vi "Get Plot at Mouse Click in Plot Area [CA].vi"(8 "error in (no error)":errorcluster, 10 "Mouse Click Coordinates":T1, 11 "XY Graph":refnum<vi>) -> (0 "error out":errorcluster, 1 "Plot Index":i32, 3 "XY Graph":refnum<vi>)   [LabVIEW 2021, in "Graphs.lvlib"]
uses:
  Graphs.lvlib
  <vilib>/Utility/miscctls.llb/LVPoint32TypeDef.ctl
panel:
  in  "Array of Complex Numbers":cdb[](array[numeric])
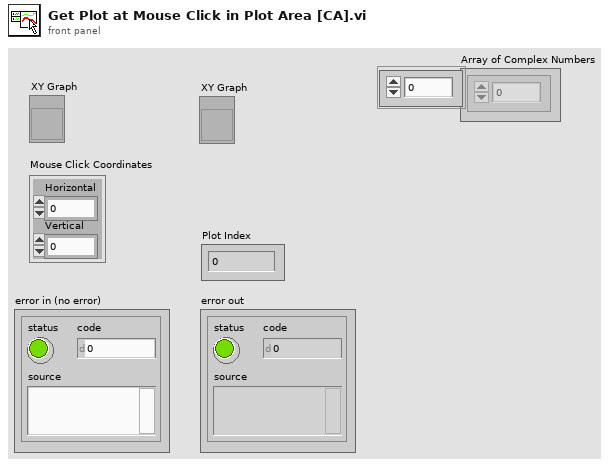
[diagram p1: front panel]
types:
  T1 = typedef "LVPoint32TypeDef.ctl" = cluster{"Horizontal":i32, "Vertical":i32}
  T2 = typedef "LVRectTypeDef.ctl" = cluster{"Left":i16, "Top":i16, "Right":i16, "Bottom":i16}
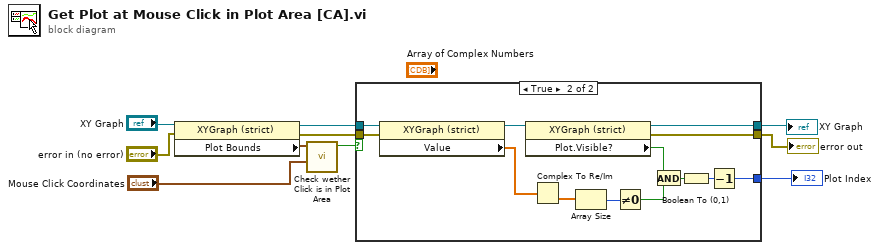
[diagram p0: block diagram]
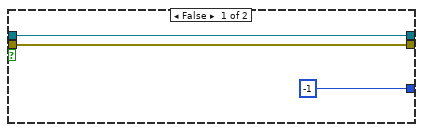
[diagram p2: hidden frame]
diagram:
  n1 = property class="XYGraph (strict)"(reference="XY Graph", error in="error in (no error)") -> (reference out=w6:refnum<vi>, error out=w7:errorcluster, "Plot Bounds"=w1:T2)
  n2 = call "Check wether Click is in Plot Area.vi"("Mouse Click Coordinates"="Mouse Click Coordinates", "Plot Bounds"=w1) -> ("Is in Plot Area?"=w8:bool)  [unwired: 8 in, 1 out]
  n3 = case shown="True" w8 {
    tunnel: w7 -> [w12 w22]
    tunnel: w6 -> [w13 w26]
    tunnel: [w13 w24] -> w5
    tunnel: [w12 w14] -> w4
    tunnel: [-1 ("Plot Index") w15] -> w3
    frame False {
    }
    frame True {
      n4 = property class="XYGraph (strict)"(reference=w26, error in=w22) -> (reference out=w25:refnum<vi>, "Value"=w23:cdb[])  [unwired: 1 out]
      n5 = property class="XYGraph (strict)"(reference=w25) -> (reference out=w24:refnum<vi>, error out=w14:errorcluster, "Plot.Visible?"=w19:bool)  [unwired: 1 in]
      n6 = Complex To Re/Im(x + iy=w23) -> (y=w21:dbl[])  [unwired: 1 out]
      n7 = Array Size(array=w21) -> (size(s)=w20:i32)
      n8 = Not Equal To 0?(x=w20) -> (x != 0?=w18:bool)
      n9 = And(x=w19, y=w18) -> (x .and. y?=w17:bool)
      n10 = Boolean To (0,1)(Boolean=w17) -> (0, 1=w16:i16)
      n11 = Decrement(x=w16) -> (x-1=w15:i16)
    }
  }
  "Plot Index" <- w3
  "XY Graph" <- w5
  "error out" <- w4
